vi "Modbus Global (slave).vi"(0 "HMI Coil":T2, 1 "Modbus Mode (Write Coil)":T3=enum."Write Coil", 5 "HMI Reg":T1, 7 "Coil IN":bool, 9 "Reg Data IN":u16, 11 "Error IN":errorcluster) -> (4 "Coils OUT":bool[](array[boolean]), 6 "Registers OUT":u16[](array[numeric]), 15 "Error OUT":errorcluster)   [LabVIEW 2020]
uses:
  Type Defs/Modbus Mode.ctl
  Type Defs/HMI Coils.ctl
  Type Defs/HMI Registers.ctl
  <vilib>/Modbus/slave/Modbus Slave.lvclass
  <vilib>/Modbus/slave/Create Slave Instance (TCP).vi
  <vilib>/Modbus/slave/Create Slave Instance (Serial).vi
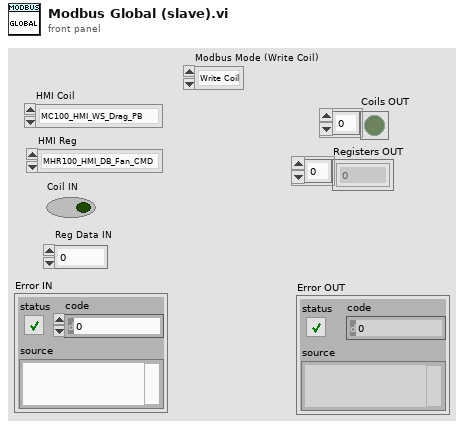
[diagram p1: front panel]
types:
  T1 = typedef "HMI Registers.ctl" = enum16{"MHR100_HMI_DB_Fan_CMD", "MHR101_HMI_DB_Drag_CMD", "MHR102_HMI_DB_TF_CMD", "MHR103_HMI_U_Trough_CMD", "MHR104_HMI_Leg_CMD", "MHR105_HMI_VFD_Select"}
  T2 = typedef "HMI Coils.ctl" = enum16{"MC100_HMI_WS_Drag_PB", "MC101_HMI_WB_Drag_PB", "MC102_HMI_WS_Fan_PB", "MC103_HMI_WB_Fan_PB", "MC104_HMI_Dryr_Drag_PB", "MC105_HMI_Dryr_Fan_PB", "MC106_HMI_DB_Fan_PB", "MC107_HMI_DB_Drag_PB", "MC108_HMI_DB_Top_Feed_PB", "MC109_HMI_U-Trough_PB", "MC110_HMI_Leg_PB", "MC111", "MC112", "MC113", "MC114", "MC115", "MC116", "MC117", "MC118", "MC119", "MC220_HMI_VFD_+100_PB", "MC221_HMI_VFD_+10_PB", "MC222_HMI_VFD_-10_PB", "MC223_HMI_VFD_-100_PB"}
  T3 = typedef "Modbus Mode.ctl" = enum16{"Init", "Read", "Write Coil", "Write Reg", "Close"}
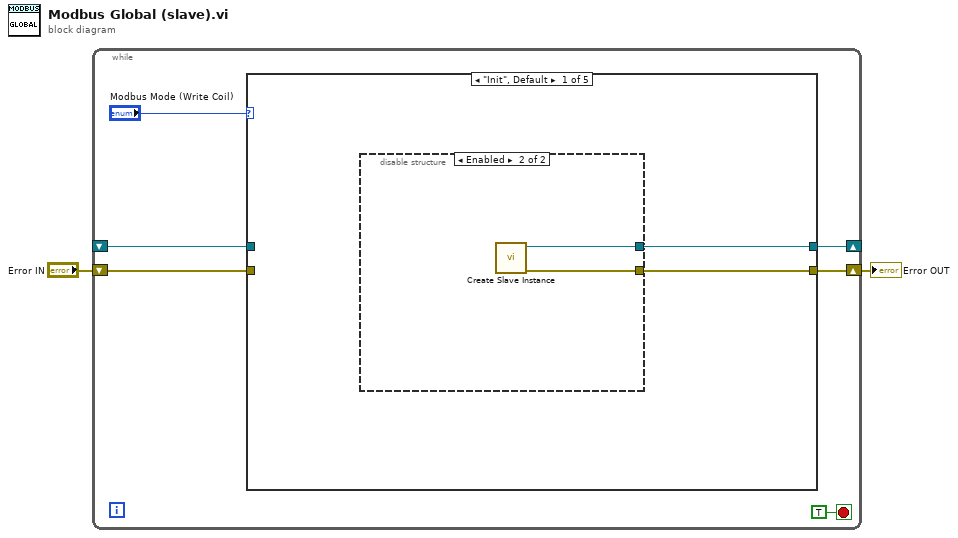
[diagram p0: block diagram]
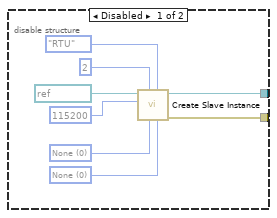
[diagram p2: hidden frame]
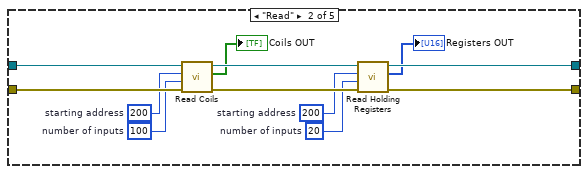
[diagram p3: hidden frame]
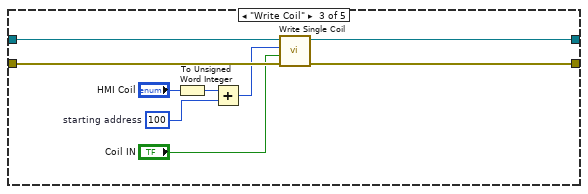
[diagram p4: hidden frame]
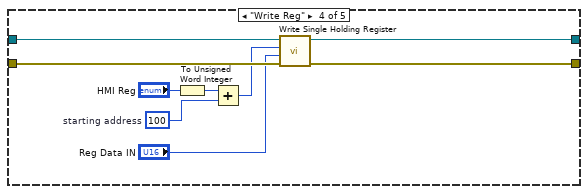
[diagram p5: hidden frame]
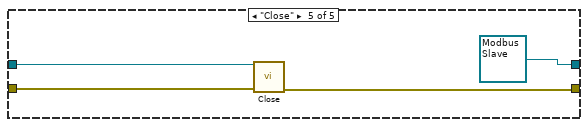
[diagram p6: hidden frame]
diagram:
  n1 = while {
    shift-right: [w6] -> _
    shift-left: _ -> [w4]
    shift-right: [w5] -> w1
    shift-left: "Error IN" -> [w3]
    stop <- TRUE stop-if-true
    n2 = case shown="\"Init\", Default" "Modbus Mode (Write Coil)" {
      tunnel: [w10 w28 w39 w48 refnum<class "Modbus Slave.lvclass"> refnum ("serial slave instance")] -> w6
      tunnel: [w9 w27 w38 w47 w52] -> w5
      tunnel: w4 -> [_ w32 w41 w50 w54]
      tunnel: w3 -> [_ w31 w40 w49 w53]
      frame "Init", Default {
        n3 = disable-structure shown="Enabled" {
          disable-tunnel: [w15 w20] -> w10
          disable-tunnel: [w14 w19] -> w9
          frame Disabled {
            w18 = u16 0 items=["None", "XON/XOFF", "RTS/CTS", "XON/XOFF & RTS/CTS", "DTR/DSR", "XON/XOFF & DTR/DSR"] ("flow control")
            w11 = u16 0 items=["None", "Odd", "Even", "Mark", "Space"] ("parity (even)")
            n4 = call-poly <vilib>:"Create Slave Instance.vi"("flow control (None)"=w18, "serial type"=enum16{"RTU", "ASCII"}."RTU", "parity (Even)"=w11, "unit ID"=u8 2, "baud rate (9600)"=u32 115200, "VISA resource name"=refnum<visa-resource-name> "COM3") -> ("error out"=w14:errorcluster, "serial slave instance"=w15:refnum<class "Modbus Slave.lvclass">)  [unwired: 4 in]
          }
          frame Enabled {
            n5 = call-poly <vilib>:"Create Slave Instance.vi"() -> ("error out"=w19:errorcluster, "TCP slave instance"=w20:refnum<class "Modbus Slave.lvclass">)  [unwired: 10 in]
          }
        }
      }
      frame "Read" {
        w22 = u16 20  # number of inputs
        w23 = u16 200  # starting address
        w25 = u16 100  # number of inputs
        w26 = u16 200  # starting address
        n6 = call-dynamic "Read Coils.vi"("error in (no error)"=w31, "number of coils"=w25, "starting address"=w26, "Modbus slave in"=w32) -> ("error out"=w29:errorcluster, "coil values"=→"Coils OUT":bool[], "Modbus slave out"=w30:refnum<class "Modbus Slave.lvclass">)  [unwired: 5 in]
        n7 = call-dynamic "Read Holding Registers.vi"("error in (no error)"=w29, "number of holding registers"=w22, "starting address"=w23, "Modbus slave in"=w30) -> ("error out"=w27:errorcluster, "register values"=→"Registers OUT":u16[], "Modbus slave out"=w28:refnum<class "Modbus Slave.lvclass">)  [unwired: 5 in]
      }
      frame "Write Coil" {
        w36 = u16 100  # starting address
        n8 = To Unsigned Word Integer(number="HMI Coil") -> (unsigned 16bit integer=w35:u16)
        n9 = Add(x=w35, y=w36) -> (x+y=w34:u16)
        n10 = call-dynamic "Write Single Coil.vi"("error in (no error)"=w40, "coil value"="Coil IN", "address"=w34, "Modbus slave in"=w41) -> ("error out"=w38:errorcluster, "Modbus slave out"=w39:refnum<class "Modbus Slave.lvclass">)  [unwired: 6 in]
      }
      frame "Write Reg" {
        w45 = u16 100  # starting address
        n11 = To Unsigned Word Integer(number="HMI Reg") -> (unsigned 16bit integer=w44:u16)
        n12 = Add(x=w44, y=w45) -> (x+y=w43:u16)
        n13 = call-dynamic "Write Single Holding Register.vi"("error in (no error)"=w49, "holding register value"="Reg Data IN", "address"=w43, "Modbus slave in"=w50) -> ("error out"=w47:errorcluster, "Modbus slave out"=w48:refnum<class "Modbus Slave.lvclass">)  [unwired: 6 in]
      }
      frame "Close" {
        n14 = call-dynamic "Close.vi"("error in (no error)"=w53, "Modbus slave in"=w54) -> ("error out"=w52:errorcluster)  [unwired: 9 in]
      }
    }
  }
  "Error OUT" <- w1
